vi "If statement Structure given index handler.vi"(8 "end index":i32, 9 "else index":i32, 10 "function true?":bool, 11 "Auto Scripting array in":T1) -> (3 "Auto Scripting array out":T1)   [LabVIEW 2013]
uses:
  Autonmous Scripting array typedef.ctl
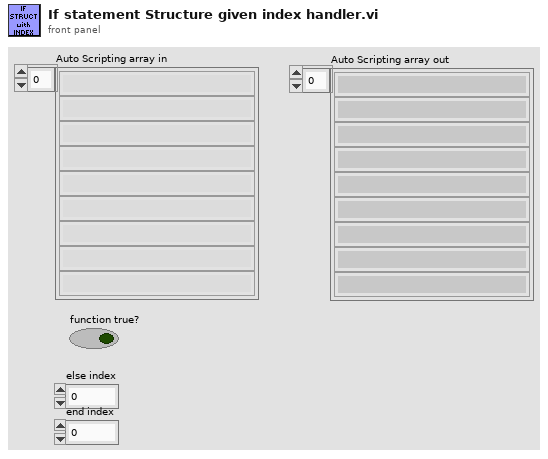
[diagram p1: front panel]
types:
  T1 = typedef "Autonmous Scripting array typedef.ctl" = string[]
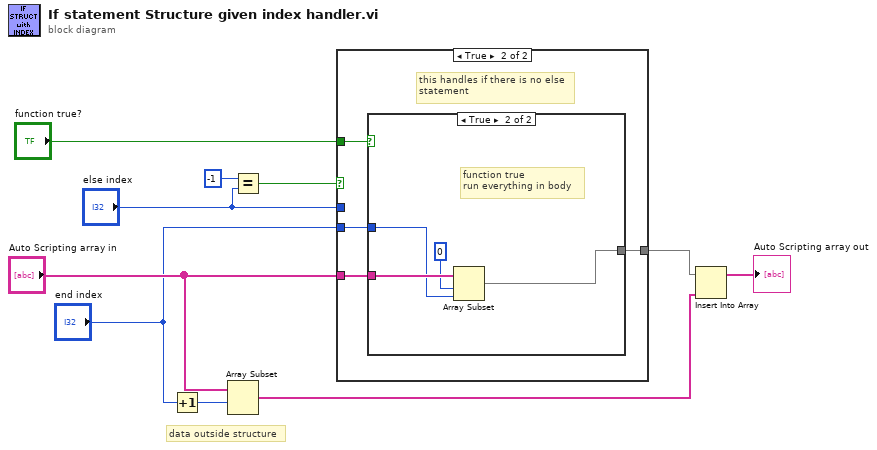
[diagram p0: block diagram]
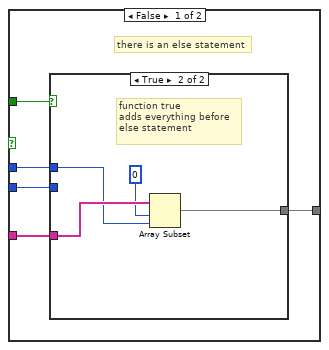
[diagram p2: hidden frame]
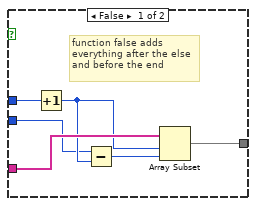
[diagram p3: hidden frame]
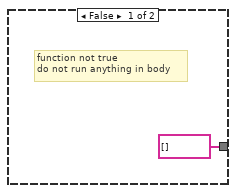
[diagram p4: hidden frame]
diagram:
  # "data outside structure"
  n1 = Increment(x="end index") -> (x+1=w1:i32)
  n2 = Array Subset(array="Auto Scripting array in", index=w1) -> (w6:T1)  [unwired: 1 in]
  n3 = Equal?(x=-1, y="else index") -> (x = y?=w9:bool)
  n4 = case shown="True" w9 {
    tunnel: "function true?" -> [w15 w29]
    tunnel: "end index" -> [w14 w27]
    tunnel: "Auto Scripting array in" -> [w13 w28]
    tunnel: "else index" -> [w12 _]
    tunnel: [w11 w26] -> w5
    frame False {
      # "there is an else statement"
      n5 = case shown="True" w15 {
        tunnel: w14 -> [w16 _]
        tunnel: w13 -> [w21 w25]
        tunnel: w12 -> [w20 w22]
        tunnel: [w18 w23] -> w11
        frame False {
          # "function false adds\neverything after the else\nand before the end"
          n6 = Increment(x=w20) -> (x+1=w17:i32)
          n7 = Subtract(x=w16, y=w17) -> (x-y=w19:i32)
          n8 = Array Subset(array=w21, index=w17, length=w19) -> (w18:T1)
        }
        frame True {
          # "function true\nadds everything before\nelse statement"
          n9 = Array Subset(array=w25, index=0, length=w22) -> (w23:T1)
        }
      }
    }
    frame True {
      # "this handles if there is no else\nstatement"
      n10 = case shown="True" w29 {
        tunnel: w28 -> [_ w34]
        tunnel: w27 -> [_ w31]
        tunnel: [T1 [] w32] -> w26
        frame False {
          # "function not true\ndo not run anything in body"
        }
        frame True {
          # "function true\nrun everything in body"
          n11 = Array Subset(array=w34, index=0, length=w31) -> (w32:T1)
        }
      }
    }
  }
  n12 = Insert Into Array(array=w5, new element=w6) -> (→"Auto Scripting array out":T1)  [unwired: 1 in]
